vi "Decode messages - remove.vi"() -> ()   [LabVIEW 2025]
panel:
  out "Numeric test data":i32
  out "String test data":string
  in  "Correct answer":bool
  in  "Communication":T1(array[cluster])
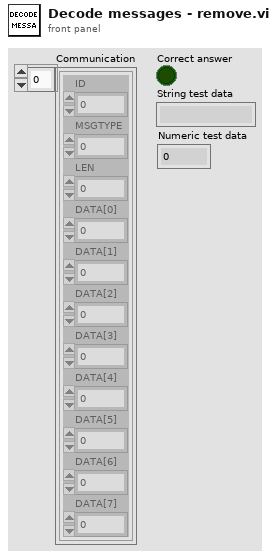
[diagram p1: front panel]
types:
  T1 = cluster{"ID":u32, "MSGTYPE":u8, "LEN":u8, "DATA[0]":u8, "DATA[1]":u8, "DATA[2]":u8, "DATA[3]":u8, "DATA[4]":u8, "DATA[5]":u8, "DATA[6]":u8, "DATA[7]":u8}[]
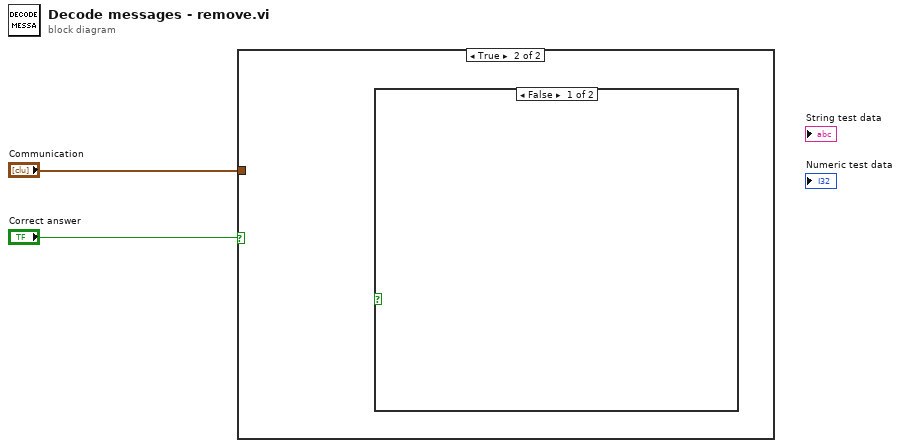
[diagram p0: block diagram]
diagram:
  n1 = case shown="True" "Correct answer" {
    tunnel: "Communication" -> [_ _]
    frame False {
    }
    frame True {
      n2 = case shown="False" {
        selector: _ -> [_ _]
        frame False {
        }
        frame True {
        }
      }
    }
  }
